vi "FFT_Summary_to_String.vi"(9 "# peaks to report":i32=3, 10 "df":dbl=0.07322788517867605, 11 "Power Spectrum (V^2 rms)":dbl[](array[numeric])=array[5121 elements]) -> (2 "Data":string[](array[string]), 3 "Header":string[](array[string]))   [LabVIEW 2016]
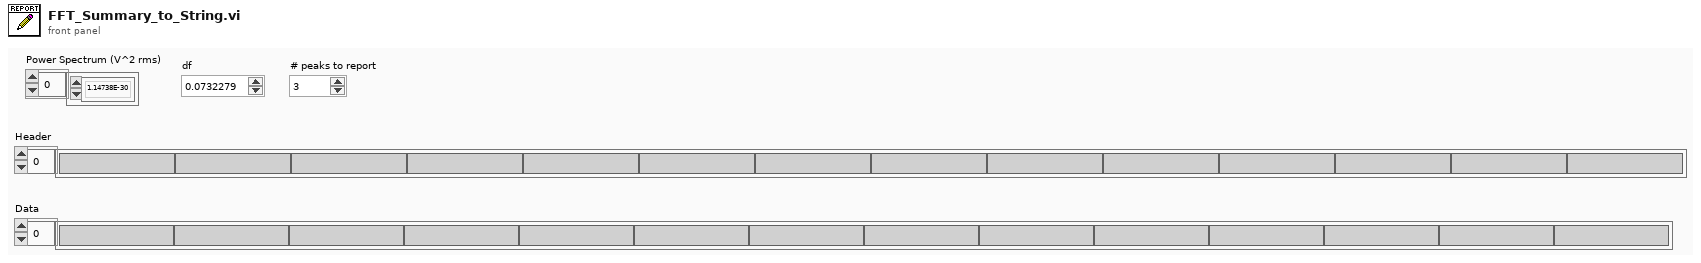
[diagram p1: front panel]
types:
  T1 = cluster{"Power (dB)":dbl, "Peak freq (Hz)":dbl}[]
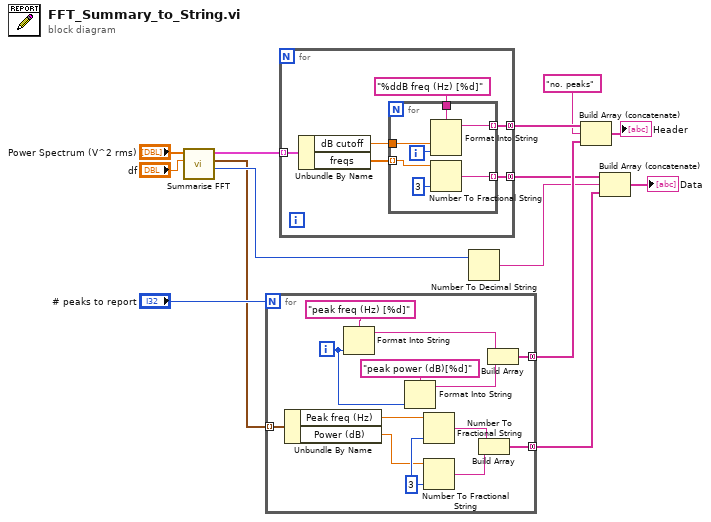
[diagram p0: block diagram]
diagram:
  n1 = call "Summarise FFT.vi"("df"="df", "Power Spectrum (V^2 rms)"="Power Spectrum (V^2 rms)") -> ("peaks found"=w3:i32, "Dominant freqs"=w1:T1, "Cuttoff freqs"=w14:cluster{"dB cutoff":dbl, "freqs":dbl[]}[])  [unwired: 7 in]
  n2 = for {
    N: "# peaks to report" -> [_]
    tunnel: [w22] -> w9 mode=concatenating
    tunnel: [w18] -> w5 mode=concatenating
    tunnel: w1 -> [w17] mode=indexing
    i -> [w25]
    w21 = i16 3 ("precision (6)")
    n3 = Unbundle By Name(w17) -> ("Peak freq (Hz)"=w16:dbl, "Power (dB)"=w15:dbl)
    n4 = Format Into String(format string="peak freq (Hz) [%d]", w25) -> (resulting string=w23:string)  [unwired: 2 in, 1 out]
    n5 = Format Into String(format string="peak power (dB)[%d]", w25) -> (resulting string=w24:string)  [unwired: 2 in, 1 out]
    n6 = Number To Fractional String(number=w16, precision (6)=w21) -> (F-format string=w20:string)  [unwired: 2 in]
    n7 = Number To Fractional String(number=w15, precision (6)=w21) -> (F-format string=w19:string)  [unwired: 2 in]
    n8 = Build Array(w20, w19) -> (w18:string[])
    n9 = Build Array(w23, w24) -> (w22:string[])
  }
  n10 = for {
    tunnel: w14 -> [w33] mode=indexing
    tunnel: [w29] -> w10 mode=concatenating
    tunnel: [w28] -> w8 mode=concatenating
    n11 = Unbundle By Name(w33) -> ("dB cutoff"=w31:dbl, "freqs"=w30:dbl[])
    n12 = for {
      tunnel: "%ddB freq (Hz) [%d]" ("format string") -> [w40]
      tunnel: w31 -> [w39]
      tunnel: w30 -> [w38] mode=indexing
      tunnel: [w35] -> w29 mode=indexing
      tunnel: [w34] -> w28 mode=indexing
      i -> [w36]
      n13 = Format Into String(format string=w40, w39, w36) -> (resulting string=w35:string)  [unwired: 2 in, 1 out]
      n14 = Number To Fractional String(number=w38, precision (6)=i16 3) -> (F-format string=w34:string)  [unwired: 2 in]
    }
  }
  n15 = Number To Decimal String(number=w3) -> (decimal integer string=w2:string)  [unwired: 1 in]
  n16 = Build Array (concatenate)(w10, "no. peaks", w9) -> (→"Header":string[])
  n17 = Build Array (concatenate)(w8, w2, w5) -> (→"Data":string[])
